vi "tm_opencamera.vi"(7 "Force Open":bool, 8 "error in (no error)":errorcluster {"code" format="%.0x"}, 11 "Camera Index":u32) -> (0 "error out":errorcluster {"code" format="%.0x"}, 3 "Handle out":u32)   [LabVIEW 2012]
uses:
  tmcamcon.dll
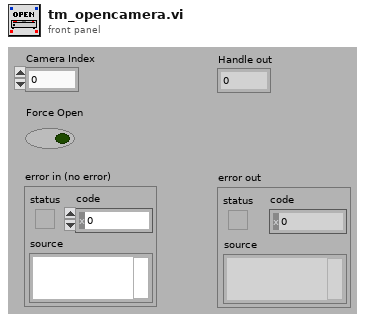
[diagram p1: front panel]
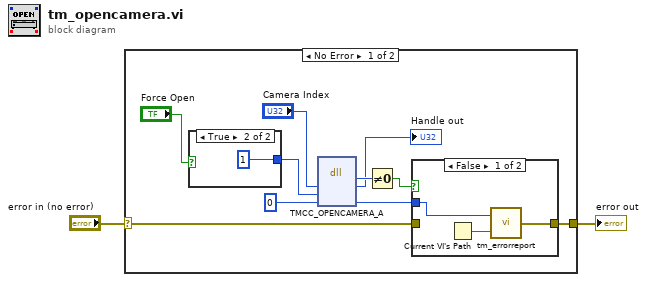
[diagram p0: block diagram]
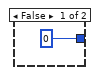
[diagram p3: hidden frame]
diagram:
  n1 = case shown="No Error" "error in (no error)" {
    selector: "error in (no error)" -> [w6 w19]
    tunnel: [w5 w19] -> w1
    frame No Error {
      n2 = case shown="True" "Force Open" {
        tunnel: [0 1] -> w7
        frame False {
        }
        frame True {
        }
      }
      n3 = dll-call lib="tmcamcon.dll" fn="TMCC_OPENCAMERA_A"("i"="Camera Index", "force"=w7, "Erval"=0) -> ("return type"=w12:u32, "i"=→"Handle out":u32, "Erval"=w4:i32)  [unwired: 4 in, 2 out]
      n4 = Not Equal To 0?(x=w12) -> (x != 0?=w3:bool)
      n5 = case shown="False" w3 {
        tunnel: w6 -> [_ w16]
        tunnel: [w14 w16] -> w5
        tunnel: w4 -> [w13 _]
        frame False {
          n6 = Current VI's Path() -> (path=w15:path)
          n7 = call <userlib>:"tm_errorreport.vi"("Source"=w15, "Error"=w13) -> ("error out"=w14:errorcluster)
        }
        frame True {
        }
      }
    }
    frame Error {
    }
  }
  "error out" <- w1
